vi "Projekt_KSP(SubVI).vi"() -> (3 "array":i32[][](array[numeric]))   [LabVIEW 2020]
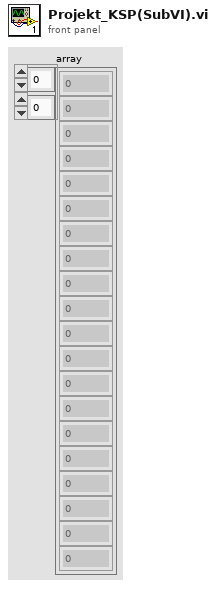
[diagram p1: front panel]
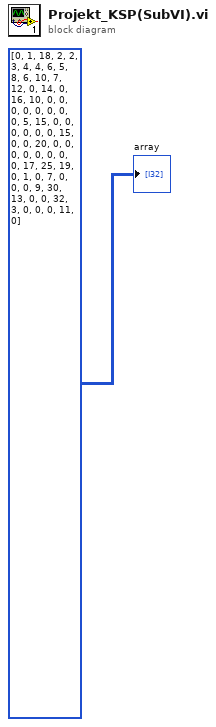
[diagram p0: block diagram]
diagram:
  "array" <- i32[][] [[0, 1], [18, 2], [2, 3], [4, 4], [6, 5], [8, 6], [10, 7], [12, 0], [14, 0], [16, 10], [0, 0], [0, 0], [0, 0], [0, 0], [5, 15], [0, 0], [0, 0], [0, 0], [15, 0], [0, 20], [0, 0], [0, 0], [0, 0], [0, 0], [17, 25], [19, 0], [1, 0], [7, 0], [0, 0], [9, 30], [13, 0], [0, 32], [3, 0], [0, 0], [11, 0]] ("array")
